vi "Adjust Color Image.vi"(8 "error in (no error)":errorcluster, 11 "24-bit pixmap":u32[][](array[numeric]) format="%x") -> (0 "error out":errorcluster, 2 "Blue Image":u32[][](array[numeric]))   [LabVIEW 2011]
doc: "This VI will take <B>Image Data in</B> and create <B>Image Data out</B> which is the same image with 50% transparency from the original. This will make the image appear greyed out or disabled. Note that this function only works with images that have opacity in the image data like 32Bit images. If the image data is not 32Bit it will be converted to it with the assumption that all pixels are solid."
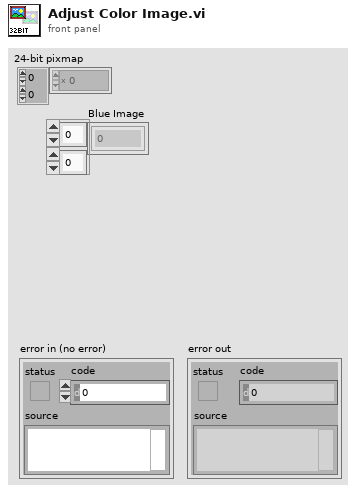
[diagram p1: front panel]
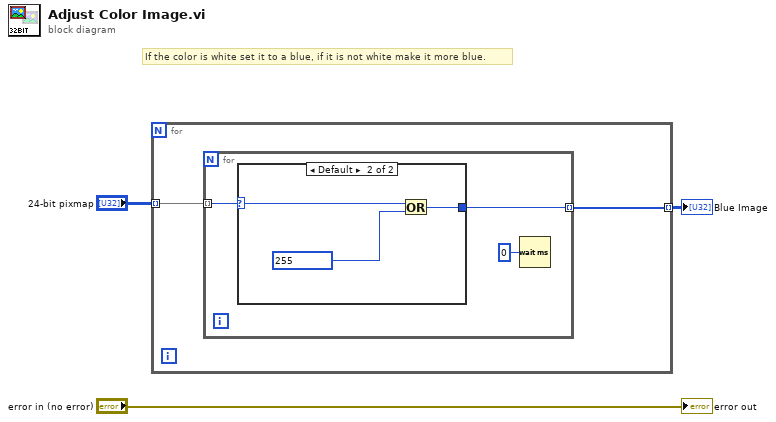
[diagram p0: block diagram]
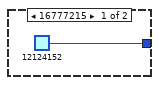
[diagram p2: hidden frame]
diagram:
  # "If the color is white set it to a blue, if it is not white make it more blue."
  n1 = for {
    tunnel: "24-bit pixmap" -> [w5] mode=indexing
    tunnel: [w4] -> w1 mode=indexing
    n2 = for {
      tunnel: w5 -> [w6] mode=indexing
      tunnel: [w8] -> w4 mode=indexing
      n3 = case shown="Default" w6 {
        selector: w6 -> [_ w10]
        tunnel: [u32 12124152 w11] -> w8
        frame 16777215 {
        }
        frame Default {
          n4 = Or(x=w10, y=u32 255) -> (x .or. y?=w11:u32)
        }
      }
      n5 = Wait (ms)(milliseconds to wait=u32 0) -> ()  [unwired: 1 out]
    }
  }
  "Blue Image" <- w1
  "error out" <- "error in (no error)"
